vi "Define Custom Glyphs by Extension.vi"(8 "error in (no error)":errorcluster, 11 "Test Executive Explorer in":refnum<class "Test Executive Explorer.lvclass">) -> (0 "error out":errorcluster, 3 "Test Executive Explorer out":refnum<class "Test Executive Explorer.lvclass">)   [LabVIEW 2019, in "Test Executive Explorer.lvclass"]
uses:
  <vilib>/gpm_packages/@cs/Test-executive-builder/Example/Application/Test Executive Explorer/Test Executive Explorer/Test Executive Explorer.lvclass
  C:/Program Files/National Instruments/LabVIEW 2019/vi.lib/gpm_packages/@cs/file-explorer-extension/Source/File Explorer/File Explorer/File Explorer.lvclass
  <vilib>/gpm_packages/@cs/file-explorer-extension/Source/File Explorer/File Explorer/Custom Glyph Definition.ctl
  <vilib>/picture/picture.llb/imagedata.ctl
  <vilib>/gpm_packages/@cs/file-explorer-extension/Source/File Explorer/File Explorer/File Explorer.lvclass/File Explorer.ctl
  <vilib>/gpm_packages/@cs/file-explorer-extension/Source/File Explorer/File Explorer/File Explorer.lvclass
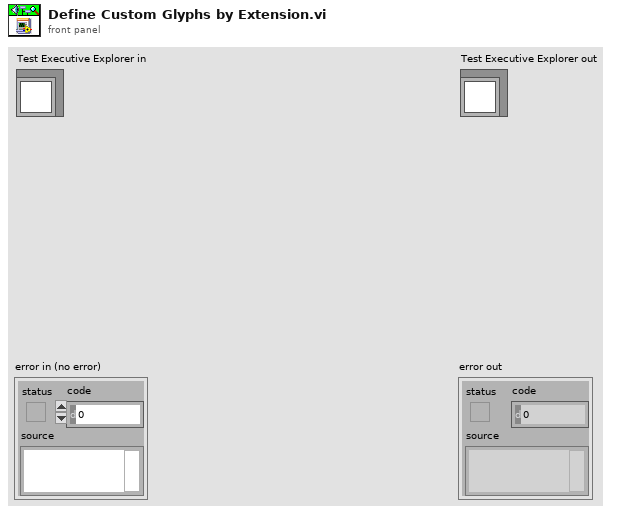
[diagram p1: front panel]
types:
  T1 = typedef "File Explorer.lvlib/File Explorer.lvclass/Custom Glyph Definition.ctl" = cluster{"Extension":string, "Glyph":T2}
  T2 = typedef "imagedata.ctl" = cluster{"image type":i32, "image depth":i32, "image":u8[], "mask":u8[], "colors":u32[], "Rectangle":cluster{"left":i16, "top":i16, "right":i16, "bottom":i16}}
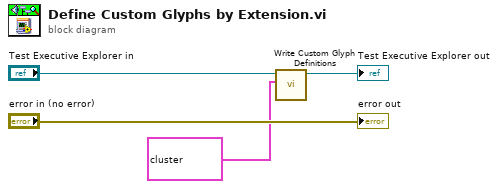
[diagram p0: block diagram]
diagram:
  n1 = call <vilib>:"Write Custom Glyph Definitions.vi"("Custom Glyph Definitions"=T1[] [{"Extension"="proc", "Glyph"={"image type"=0, "image depth"=32, "image"=array[3600 elements], "mask"=[0, 0, 0, 0, 0, 0, 0, 0, 0, 0, 0, 0, 63, 255, 255, 240, 63, 255, 255, 240, 63, 255, 255, 240, 63, 255, 255, 240, 63, 255, 255, 240, 63, 255, 255, 240, 63, 255, 255, 240, 63, 255, 255, 240, 63, 255, 255, 240, 63, 255, 255, 240, 63, 255, 255, 240, 63, 255, 255, 240, 63, 255, 255, 240, 63, 255, 255, 240, 63, 255, 255, 240, 63, 255, 255, 240, 63, 255, 255, 240, 63, 255, 255, 240, 63, 255, 255, 240, 63, 255, 255, 248, 63, 255, 255, 248, 63, 255, 255, 224, 63, 255, 255, 128, 0, 0, 127, 0, 0, 0, 124, 0, 0, 0, 112, 0, 0, 0, 64, 0], "colors"=[], "Rectangle"={"left"=0, "top"=0, "right"=30, "bottom"=30}}}, {"Extension"="tmp", "Glyph"={"image type"=0, "image depth"=32, "image"=array[3600 elements], "mask"=[0, 0, 0, 0, 0, 0, 0, 0, 0, 0, 0, 0, 63, 255, 255, 240, 127, 255, 255, 248, 127, 255, 255, 248, 127, 255, 255, 248, 127, 255, 255, 248, 127, 255, 255, 248, 127, 255, 255, 248, 127, 255, 255, 248, 127, 255, 255, 248, 127, 255, 255, 248, 127, 255, 255, 248, 127, 255, 255, 248, 127, 255, 255, 248, 127, 255, 255, 248, 127, 255, 255, 248, 127, 255, 255, 248, 127, 255, 255, 248, 127, 255, 255, 248, 127, 255, 255, 248, 127, 255, 255, 248, 127, 255, 255, 248, 127, 255, 255, 248, 127, 255, 255, 248, 127, 255, 255, 240, 0, 0, 31, 224, 0, 0, 31, 160, 0, 0, 3, 0], "colors"=[], "Rectangle"={"left"=0, "top"=0, "right"=30, "bottom"=30}}}, {"Extension"="set", "Glyph"={"image type"=0, "image depth"=32, "image"=array[3600 elements], "mask"=[0, 0, 0, 0, 0, 0, 0, 0, 0, 0, 0, 0, 63, 255, 255, 240, 63, 255, 255, 240, 63, 255, 255, 240, 63, 255, 255, 240, 63, 255, 255, 240, 63, 255, 255, 240, 63, 255, 255, 240, 63, 255, 255, 240, 63, 255, 255, 240, 63, 255, 255, 240, 63, 255, 255, 240, 63, 255, 255, 240, 63, 255, 255, 240, 63, 255, 255, 252, 63, 255, 255, 252, 63, 255, 255, 252, 63, 255, 255, 252, 63, 255, 255, 252, 63, 255, 255, 252, 63, 255, 255, 252, 63, 255, 255, 252, 63, 255, 255, 252, 63, 255, 255, 252, 0, 0, 255, 252, 0, 0, 255, 252, 0, 0, 255, 252, 0, 0, 127, 248], "colors"=[], "Rectangle"={"left"=0, "top"=0, "right"=30, "bottom"=30}}}], "File Explorer in"="Test Executive Explorer in") -> ("File Explorer out"=→"Test Executive Explorer out":refnum<class "Test Executive Explorer.lvclass">)  [unwired: 9 in]
  "error out" <- "error in (no error)"
